vi "convert_step_vs_opening.vi"(8 "bypass_valve_opening_in":dbl, 9 "bypass_valve_step_in":i32, 10 "run_valve_opening_in":dbl, 11 "run_valve_step_in":i32) -> (0 "bypass_valve_step_out":i32, 1 "bypass_valve_opening_out":dbl, 2 "run_valve_step_out":i32, 3 "run_valve_opening_out":dbl)   [LabVIEW 2019]
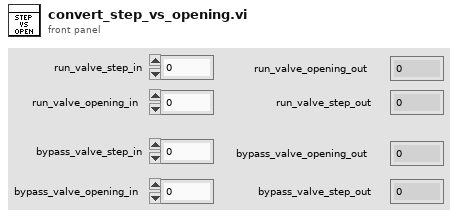
[diagram p1: front panel]
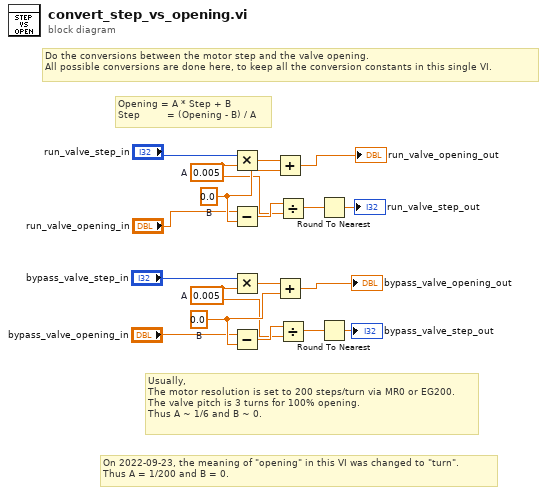
[diagram p0: block diagram]
diagram:
  w8 = 0.0  # B
  w6 = 0.005  # A
  w15 = 0.0  # B
  w12 = 0.005  # A
  # "On 2022-09-23, the meaning of \"opening\" in this VI was changed to \"turn\".\nThus A = 1/200 and B = 0."
  # "Usually,\nThe motor resolution is set to 200 steps/turn via MR0 or EG200.\nThe valve pitch is 3 turns for 100% opening.\nThus A ~ 1/6 and B ~ 0."
  # "Opening = A * Step + B\nStep         = (Opening - B) / A"
  # "Do the conversions between the motor step and the valve opening.\nAll possible conversions are done here, to keep all the conversion constants in this single VI."
  n1 = Multiply(x="run_valve_step_in", y=w12) -> (x*y=w17:dbl)
  n2 = Subtract(x="run_valve_opening_in", y=w15) -> (x-y=w13:dbl)
  n3 = Multiply(x="bypass_valve_step_in", y=w6) -> (x*y=w9:dbl)
  n4 = Subtract(x="bypass_valve_opening_in", y=w8) -> (x-y=w7:dbl)
  n5 = Add(x=w17, y=w15) -> (x+y=→"run_valve_opening_out":dbl)
  n6 = Add(x=w9, y=w8) -> (x+y=→"bypass_valve_opening_out":dbl)
  n7 = Divide(x=w13, y=w12) -> (x/y=w10:dbl)
  n8 = Divide(x=w7, y=w6) -> (x/y=w5:dbl)
  n9 = Round To Nearest(number=w10) -> (nearest integer value=→"run_valve_step_out":dbl)
  n10 = Round To Nearest(number=w5) -> (nearest integer value=→"bypass_valve_step_out":dbl)
